vi "Register for Plugin Subpanel Events.vi"(7 "Plugin Subpanel Events":T1, 8 "error in (no error)":errorcluster, 11 "CIF_UI in":refnum<class "CIF_UI.lvclass">) -> (0 "error out":errorcluster, 3 "Event Registration Refnum":refnum<event-registration>)   [LabVIEW 2021, in "CIF_UI.lvclass"]
uses:
  CIF_UI.lvclass
  Typedef/Plugin Subpanel Events.ctl
  Typedef/New Connection Event Data.ctl
  <vilib>/gRPC/LabVIEW gRPC Library/Shared/grpcId.ctl
  Typedef/New Connection Plugin Event Data.ctl
  CIF_UI.lvclass/CIF_UI.ctl
  <vilib>/gRPC/LabVIEW gRPC Library/grpc-lvsupport-release.lvlib
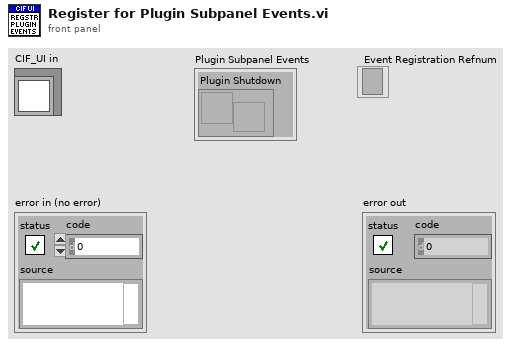
[diagram p1: front panel]
types:
  T1 = typedef "CIF_UI.lvclass/Plugin Subpanel Events.ctl" = cluster{"Plugin Shutdown":refnum<user-event>}
  T2 = typedef "CIF_UI.lvclass/SubPanel Events.ctl" = cluster{"Clear Local Error":refnum<user-event>, "Shutdown":refnum<user-event>, "gRPC Connection":refnum<user-event>, "Plugin Connection":refnum<user-event>}
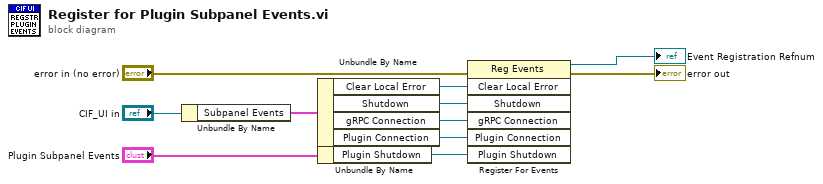
[diagram p0: block diagram]
diagram:
  n1 = Unbundle By Name("CIF_UI in") -> ("Subpanel Events"=w10:T2)
  n2 = Unbundle By Name(w10) -> ("Clear Local Error"=w9:refnum<user-event>, "Shutdown"=w8:refnum<user-event>, "gRPC Connection"=w5:refnum<user-event>, "Plugin Connection"=w4:refnum<user-event>)
  n3 = Unbundle By Name("Plugin Subpanel Events") -> ("Plugin Shutdown"=w2:refnum<user-event>)
  n4 = register-events(error in="error in (no error)", w9, w8, w5, w4, w2) -> (reference out=→"Event Registration Refnum":refnum<event-registration>, error out=→"error out":errorcluster)  [unwired: 1 in]
